vi "RemoveSideWiresFromSelectedList__slk_mt.vi"(8 "error in (no error)":errorcluster, 11 "diagram refnum in":refnum<vi>) -> (0 "error out":errorcluster, 3 "duplicated diagram refnum out":refnum<vi>)   [LabVIEW 2012, in "Lazyboots Menu Tool.lvlib"]
doc: "Removes side wires from selected list.\n\n<b>NOTE</b>: Side wire is the wires that its sourcing or sinking terminals have not been selected."
uses:
  Library/Lazyboots Menu Tool.lvlib
panel:
  # "RemoveSideWiresFromSelectedList__slk_mt.vi\nRemoves side wires from selected list.\n\nNOTICE -- YOU MUST LEAVE THIS NOTICE IN PLACE.\n\nCopyright (c) 2011, LIANG LIU Shawn.Liu.cn@gmail.com\nAll rights reserved.\n\nRedistribution and use in source and binary forms, with or without modification, are permitted provided that the following conditions are met:\n-Redistributions of source code must retain the above copyright notice, this list of conditions and the following disclaimer.\n-Redistributions in binary form must reproduce the above copyright notice, this list of conditions and the following disclaimer in the documentation and/or other materials provided with the distribution.\n-Neither the name of the eLp nor the names of its contributors may be used to endorse or promote products derived from this software without specific prior written permission.\n\nTHIS SOFTWARE IS PROVIDED BY THE COPYRIGHT HOLDERS AND CONTRIBUTORS \"AS IS\" AND ANY EXPRESS OR IMPLIED WARRANTIES, INCLUDING, BUT NOT LIMITED TO, THE IMPLIED WARRANTIES OF MERCHANTABILITY AND FITNESS FOR A PARTICULAR PURPOSE ARE DISCLAIMED. IN NO EVENT SHALL THE COPYRIGHT HOLDER OR CONTRIBUTORS BE LIABLE FOR ANY DIRECT, INDIRECT, INCIDENTAL, SPECIAL, EXEMPLARY, OR CONSEQUENTIAL DAMAGES (INCLUDING, BUT NOT LIMITED TO, PROCUREMENT OF SUBSTITUTE GOODS OR SERVICES; LOSS OF USE, DATA, OR PROFITS; OR BUSINESS INTERRUPTION) HOWEVER CAUSED AND ON ANY THEORY OF LIABILITY, WHETHER IN CONTRACT, STRICT LIABILITY, OR TORT (INCLUDING NEGLIGENCE OR OTHERWISE) ARISING IN ANY WAY OUT OF THE USE OF THIS SOFTWARE, EVEN IF ADVISED OF THE POSSIBILITY OF SUCH DAMAGE."
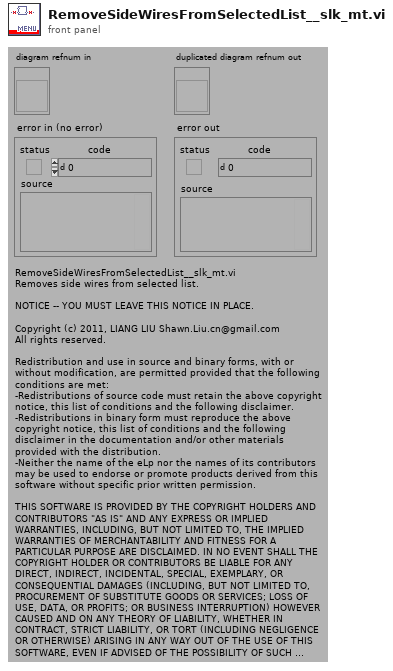
[diagram p1: front panel]
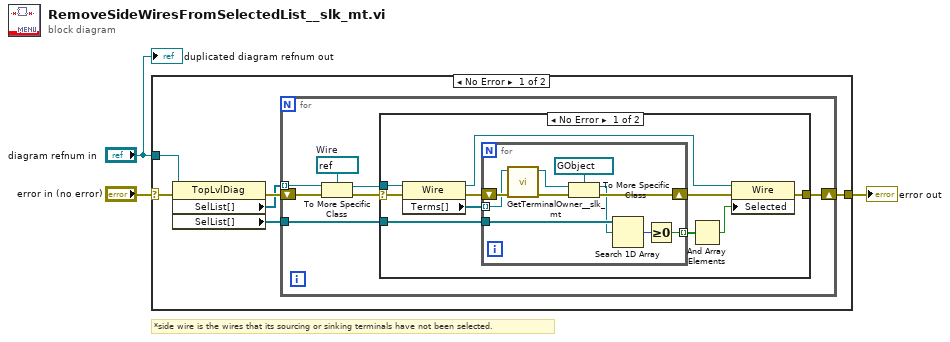
[diagram p0: block diagram]
diagram:
  # "*side wire is the wires that its sourcing or sinking terminals have not been selected."
  n1 = case shown="No Error" "error in (no error)" {
    selector: "error in (no error)" -> [w4 w37]
    tunnel: "diagram refnum in" -> [w5 _]
    tunnel: [w8 w37] -> w3
    frame No Error {
      n2 = property on="Property Node" class="TopLvlDiag"(reference=w5, error in=w4) -> (error out=w9:errorcluster, "SelList[]"=w7:refnum<vi>[], "SelList[]"=w6:refnum<vi>[])  [unwired: 1 out]
      n3 = for {
        tunnel: w7 -> [w16] mode=indexing
        tunnel: w6 -> [w14]
        shift-right: [w12] -> w8
        shift-left: w9 -> [w13]
        w10 = refnum<vi> refnum  # Wire
        n4 = To More Specific Class(target class=w10, reference=w16, error in=w13) -> (specific class reference=w15:refnum<vi>, error out=w11:errorcluster)
        n5 = case shown="No Error" w11 {
          selector: w11 -> [w17 _]
          tunnel: w15 -> [w26 _]
          tunnel: w14 -> [w24 _]
          tunnel: [w18 _] -> w12
          frame No Error {
            n6 = property class="Wire"(reference=w26, error in=w17) -> (reference out=w22:refnum<vi>, error out=w20:errorcluster, "Terms[]"=w25:refnum<vi>[])
            n7 = for {
              tunnel: w25 -> [w28] mode=indexing
              tunnel: w24 -> [w36]
              tunnel: [w33] -> w23 mode=indexing
              shift-right: [w32] -> w19
              shift-left: w20 -> [w30]
              n8 = call "GetTerminalOwner__slk_mt.vi"("error in (no error)"=w30, "terminal refnum in"=w28) -> ("error out"=w29:errorcluster, "owner refnum out"=w27:refnum<vi>)  [unwired: 3 in, 5 out]
              n9 = To More Specific Class(target class=refnum<vi> refnum ("element"), reference=w27, error in=w29) -> (specific class reference=w31:refnum<vi>, error out=w32:errorcluster)
              n10 = Search 1D Array(1D array=w36, element=w31) -> (index of element=w34:i32)  [unwired: 1 out]
              n11 = Greater Or Equal To 0?(x=w34) -> (x >= 0?=w33:bool)
            }
            n12 = And Array Elements(Boolean array=w23) -> (logical AND=w21:bool)
            n13 = property class="Wire"(reference=w22, error in=w19, "Selected"=w21) -> (error out=w18:errorcluster)  [unwired: 1 out]
          }
          frame Error {
          }
        }
      }
    }
    frame Error {
    }
  }
  "error out" <- w3
  "duplicated diagram refnum out" <- "diagram refnum in"
